vi "_RT_CtrlLoop_Pressure_Process.vi"(6 "ExpVar.lvclass":refnum<class "ExpVar.lvclass">, 8 "error in (no error)":errorcluster, 11 "RS232ComPort In":refnum<class "RS232ComPort.lvclass">) -> ()   [LabVIEW 2018]
uses:
  PublicSubVI/RS232/RS232ComPort.lvclass
  PublicSubVI/NewExpVar/ExpVar.lvclass
  PublicSubVI/Ctl/_ctl_RT_CustomCmd.ctl
  PublicSubVI/Ctl/_ctl_RT_PressureCmd.ctl
panel:
  out "Value":string
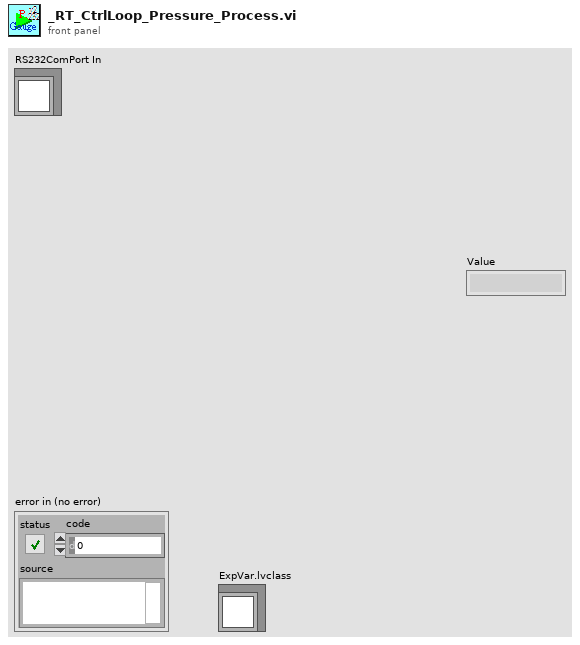
[diagram p1: front panel]
types:
  T1 = typedef "_ctl_RT_CustomCmd.ctl" = cluster{"Cmd":T2, "Value":string}
  T2 = typedef "_ctl_RT_PressureCmd.ctl" = enum8{"None", "Get_Sensor_Status", "Get_Sensor_temp", "Get_Address", "Get_BaudRate", "Get_PR1", "Get_PR4", "Get_Relay1_State", "Get_Relay2_State", "Get_Relay3_State", "Get_Switch1_Value", "Get_Switch2_Value", "Get_Switch3_Value", "Get_Enable1_State", "Get_Enable2_State", "Get_Enable3_State", "Get_Unit", "Get_Calib_Gas", "Get_Vacuum_Adj", "Get_Atmospheric_Adj", "Get_Analog_Volt1", "Get_Analog_Volt2", "Set_Address", "Set_BaudRate", "Set_Switch1_Value", "Set_Switch2_Value", "Set_Switch3_Value", "Set_Enable1_State", "Set_Enable2_State", "Set_Enable3_State", "Set_Unit", "Set_Calib_Gas", "Set_Vacuum_Adj", "Set_Atmospheric_Adj", "Set_Analog_Volt1", "Set_Analog_Volt2"}
  T3 = enum16{"via string label", "Laser", "Pressure", "TMP", "Script", "Signal Remarks", "ExtAO", "ExtDO", "ExtDI", "D999"}
  T4 = typedef "Semaphore RefNum" = refnum<k1>
  T5 = cluster{"Response Str":string, "VISA resource":refnum<visa-resource-name>, "DeviceExist?":bool, "semaphore":T4}
  T6 = cluster{"attention char + addr":string, "termination":string}
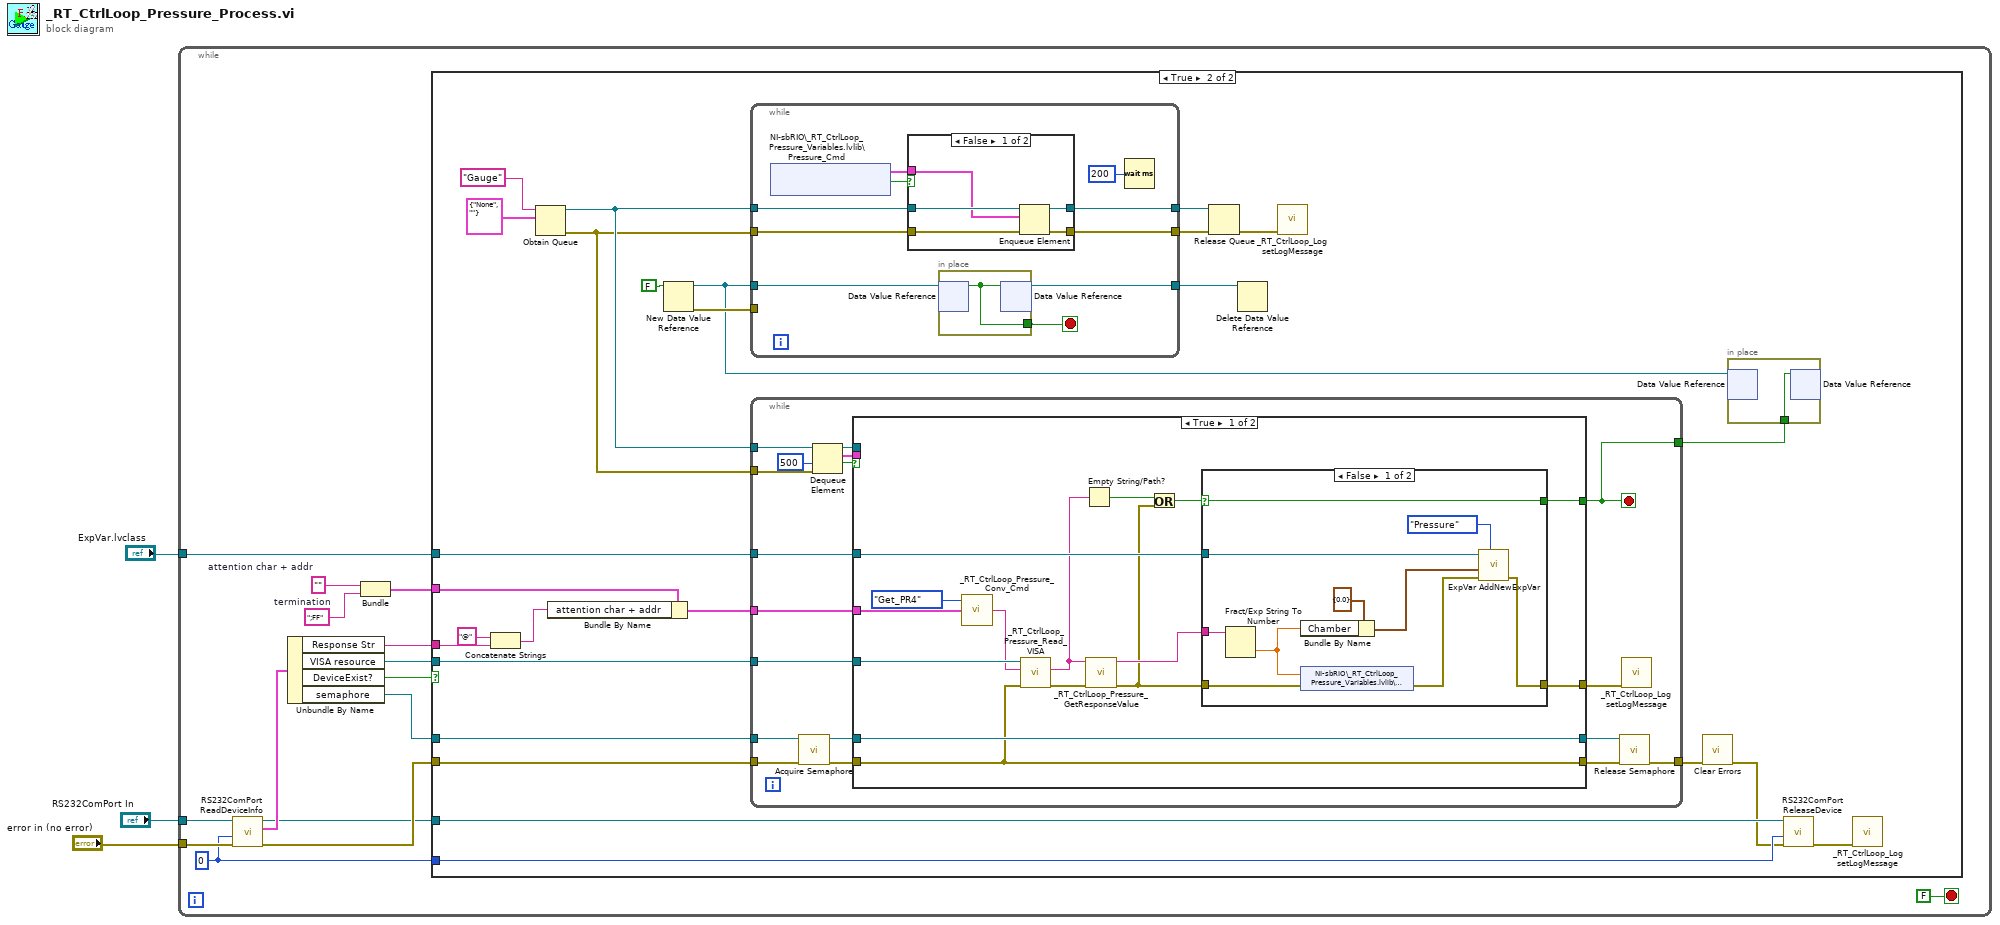
[diagram p0: block diagram]
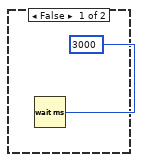
[diagram p2: hidden frame]
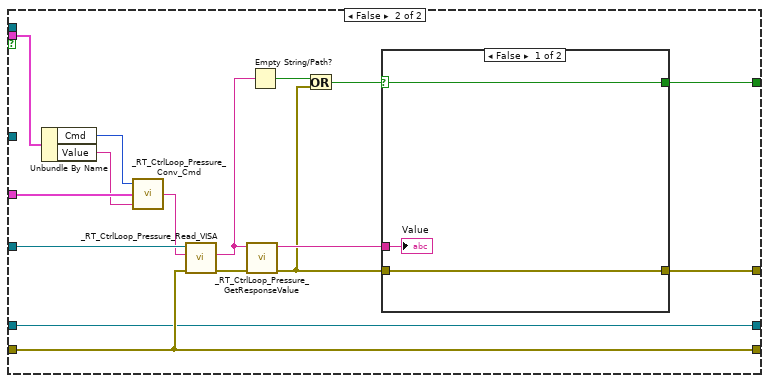
[diagram p5: hidden frame]
diagram:
  n1 = while {
    tunnel: "error in (no error)" -> [w9]
    tunnel: "RS232ComPort In" -> [w10]
    tunnel: "ExpVar.lvclass" -> [w4]
    stop <- FALSE stop-if-true
    w6 = 0
    w13 = ""  # attention char + addr
    w14 = ";FF"  # termination
    n2 = call-dynamic "RS232ComPort ReadDeviceInfo.vi"("error in (no error)"=w9, "DeviceIndex"=w6, "RS232ComPort in"=w10) -> ("error out"=w7:errorcluster, "DeviceInfo"=w8:T5, "RS232ComPort out"=w5:refnum<class "RS232ComPort.lvclass">)  [unwired: 6 in]
    n3 = Unbundle By Name(w8) -> ("Response Str"=w18:string, "VISA resource"=w17:refnum<visa-resource-name>, "DeviceExist?"=w16:bool, "semaphore"=w15:T4)
    n4 = Bundle("attention char + addr"=w13, "termination"=w14) -> (w12:T6)  [unwired: 1 in]
    n5 = case shown="True" w16 {
      tunnel: w7 -> [_ w45]
      tunnel: w18 -> [_ w43]
      tunnel: w17 -> [_ w41]
      tunnel: w15 -> [_ w39]
      tunnel: w12 -> [_ w38]
      tunnel: w6 -> [_ w34]
      tunnel: w5 -> [_ w35]
      tunnel: w4 -> [_ w33]
      frame False {
        n6 = Wait (ms)(milliseconds to wait=u32 3000) -> ()  [unwired: 1 out]
      }
      frame True {
        n7 = Concatenate Strings("@", w43) -> (w42:string)
        n8 = Obtain Queue(name (unnamed)="Gauge", element data type=T1 {"Cmd"=enum."None", "Value"=""}) -> (queue out=w37:refnum<queue>, error out=w36:errorcluster)  [unwired: 3 in, 1 out]
        n9 = Bundle By Name(cluster=w38, "attention char + addr"=w42) -> (w40:T6)
        n10 = New Data Value Reference(data value=FALSE) -> (data value reference=w21:refnum<data-value>, error out=w23:errorcluster)  [unwired: 1 in]
        n11 = while {
          tunnel: w37 -> [w56]
          tunnel: w36 -> [w55]
          tunnel: [w51] -> w28
          tunnel: [w50] -> w27
          tunnel: w21 -> [w49]
          tunnel: w23 -> [_]
          tunnel: [w47] -> w20
          stop <- w48 stop-if-true
          n12 = shared-variable "NI-sbRIO\\_RT_CtrlLoop_Pressure_Variables.lvlib\\Pressure_Cmd"() -> (w53:T1, w52:bool)  [unwired: 2 in, 1 out]
          n13 = case shown="False" w52 {
            tunnel: w56 -> [w62 w63]
            tunnel: w55 -> [w61 w64]
            tunnel: w53 -> [w60 _]
            tunnel: [w59 w64] -> w50
            tunnel: [w58 w63] -> w51
            frame False {
              n14 = Enqueue Element(queue=w62, element=w60, error in (no error)=w61) -> (queue out=w58:refnum<queue>, error out=w59:errorcluster)  [unwired: 1 in, 1 out]
            }
            frame True {
            }
          }
          n15 = in-place {
            in-place-border: [w57] -> w48
            n16 = in-place-dvr #1(w49) -> (w57:bool)  [unwired: 1 out]
            n17 = in-place-dvr #1(w57) -> (w47:refnum<data-value>)  [unwired: 1 out]
          }
          n18 = Wait (ms)(milliseconds to wait=u32 200) -> ()  [unwired: 1 out]
        }
        n19 = while {
          tunnel: w40 -> [w82]
          tunnel: w41 -> [w81]
          tunnel: w45 -> [w74]
          tunnel: w39 -> [w75]
          tunnel: w37 -> [w79]
          tunnel: w36 -> [w78]
          tunnel: [w70] -> w30
          tunnel: w33 -> [w68]
          tunnel: [w65] -> w22
          stop <- w65 stop-if-true
          n20 = call <vilib>:"Acquire Semaphore.vi"("error in (no error)"=w74, "semaphore"=w75) -> ("error out"=w72:errorcluster, "semaphore out"=w73:T4)  [unwired: 3 in, 1 out]
          n21 = Dequeue Element(queue=w79, timeout in ms (-1)=500, error in (no error)=w78) -> (queue out=w66:refnum<queue>, element=w76:T1, timed out?=w77:bool)  [unwired: 1 out]
          n22 = case shown="True" w77 {
            tunnel: w81 -> [w97 w125]
            tunnel: w82 -> [w92 w122]
            tunnel: w76 -> [_ w121]
            tunnel: w73 -> [w96 w123]
            tunnel: w72 -> [w95 w124]
            tunnel: [w96 w123] -> w71
            tunnel: [w95 w124] -> w69
            tunnel: [w94 w115] -> w67
            tunnel: w68 -> [w93 _]
            tunnel: [w83 w111] -> w65
            tunnel: w66 -> [_ _]
            frame True {
              n23 = call "_RT_CtrlLoop_Pressure_Conv_Cmd.vi"("Symbol"=w92, "Cmd"=_ctl_RT_PressureCmd."Get_PR4") -> ("Cmd String"=w91:string)  [unwired: 1 in]
              n24 = call "_RT_CtrlLoop_Pressure_Read_VISA.vi"("error in (no error)"=w95, "Comm Str"=w91, "VISA resource In"=w97) -> ("error out"=w87:errorcluster, "Response Str"=w88:string)  [unwired: 6 in, 1 out]
              n25 = Empty String/Path?(string/path=w88) -> (empty?=w86:bool)
              n26 = call "_RT_CtrlLoop_Pressure_GetResponseValue.vi"("error in"=w87, "Response Str"=w88) -> ("error out"=w84:errorcluster, "Value"=w90:string)  [unwired: 8 in]
              n27 = Or(x=w86, y=w84) -> (x .or. y?=w85:bool)
              n28 = case shown="False" w85 {
                selector: w85 -> [w98 w108]
                tunnel: w90 -> [w107 _]
                tunnel: [w102 w109] -> w94
                tunnel: w93 -> [w104 _]
                tunnel: w84 -> [w99 w109]
                tunnel: [w98 w108] -> w83
                frame False {
                  n29 = Fract/Exp String To Number(string=w107) -> (number=w106:dbl)  [unwired: 3 in, 1 out]
                  n30 = Bundle By Name(cluster=cluster{"Chamber":dbl} {"Chamber"=0.0} ("Pressure"), "Chamber"=w106) -> (w105:cluster{"Chamber":dbl})
                  n31 = shared-variable "NI-sbRIO\\_RT_CtrlLoop_Pressure_Variables.lvlib\\Pressure_dbl"(w106, error in=w99) -> (error out=w103:errorcluster)
                  n32 = call-dynamic "ExpVar AddNewExpVar.vi"("VarType"=T3."Pressure", "error in (no error)"=w103, "Var"=w105, "ExpVar in"=w104) -> ("error out"=w102:errorcluster)  [unwired: 6 in, 1 out]
                }
                frame True {
                }
              }
            }
            frame False {
              n33 = Unbundle By Name(w121) -> ("Cmd"=w120:T2, "Value"=w119:string)
              n34 = call "_RT_CtrlLoop_Pressure_Conv_Cmd.vi"("Value"=w119, "Symbol"=w122, "Cmd"=w120) -> ("Cmd String"=w118:string)
              n35 = call "_RT_CtrlLoop_Pressure_Read_VISA.vi"("error in (no error)"=w124, "Comm Str"=w118, "VISA resource In"=w125) -> ("error out"=w117:errorcluster, "Response Str"=w114:string)  [unwired: 6 in, 1 out]
              n36 = call "_RT_CtrlLoop_Pressure_GetResponseValue.vi"("error in"=w117, "Response Str"=w114) -> ("error out"=w110:errorcluster, "Value"=w116:string)  [unwired: 8 in]
              n37 = Empty String/Path?(string/path=w114) -> (empty?=w113:bool)
              n38 = Or(x=w113, y=w110) -> (x .or. y?=w112:bool)
              n39 = case shown="False" w112 {
                selector: w112 -> [w127 w130]
                tunnel: w116 -> [w128 _]
                tunnel: [w126 w129] -> w115
                tunnel: [w127 w130] -> w111
                tunnel: w110 -> [w126 w129]
                frame False {
                  "Value" <- w128
                }
                frame True {
                }
              }
            }
          }
          n40 = call <vilib>:"Release Semaphore.vi"("error in (no error)"=w69, "semaphore"=w71) -> ("error out"=w70:errorcluster)  [unwired: 4 in, 1 out]
          n41 = call "_RT_CtrlLoop_Log setLogMessage.vi"("error in"=w67) -> ()  [unwired: 9 in, 2 out]
        }
        n42 = Release Queue(queue=w28, error in (no error)=w27) -> (error out=w26:errorcluster)  [unwired: 1 in, 2 out]
        n43 = Delete Data Value Reference(data value reference=w20) -> ()  [unwired: 1 in, 2 out]
        n44 = call "_RT_CtrlLoop_Log setLogMessage.vi"("error in"=w26) -> ()  [unwired: 9 in, 2 out]
        n45 = call <vilib>:"Clear Errors.vi"("error in (no error)"=w30) -> ("error out"=w29:errorcluster)  [unwired: 5 in, 1 out]
        n46 = in-place {
          in-place-border: w22 -> [w46]
          n47 = in-place-dvr #2(w21) -> ()  [unwired: 2 out]
          n48 = in-place-dvr #2(w46) -> ()  [unwired: 2 out]
        }
        n49 = call "RS232ComPort ReleaseDevice.vi"("error in (no error)"=w29, "DeviceIndex"=w34, "RS232ComPort in"=w35) -> ("error out"=w25:errorcluster)  [unwired: 8 in]
        n50 = call "_RT_CtrlLoop_Log setLogMessage.vi"("error in"=w25) -> ()  [unwired: 9 in, 2 out]
      }
    }
  }
